vi "Get Message HasOneof.vi"(8 "error in (no error)":errorcluster, 11 "Message ref in":u64) -> (0 "error out":errorcluster, 2 "Has Oneof?":bool, 3 "Message ref out":u64)   [LabVIEW 2019, in "gRPC Template Creation Utility.lvlib"]
uses:
  gRPC Template Creation Utility.lvlib
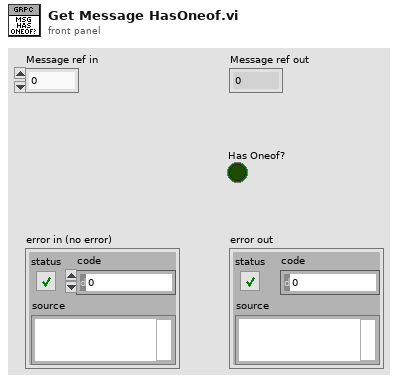
[diagram p1: front panel]
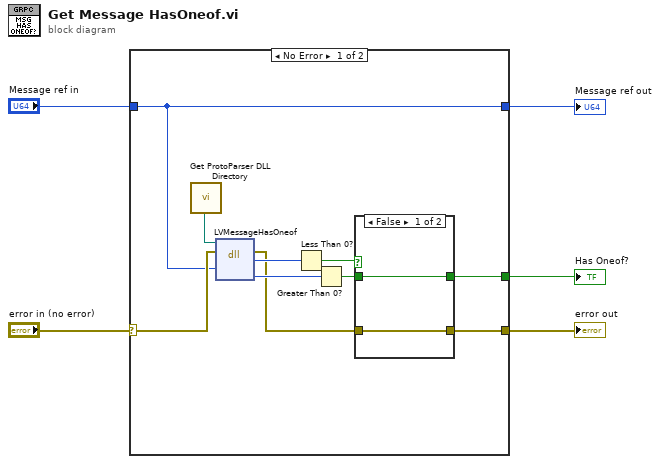
[diagram p0: block diagram]
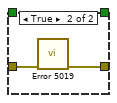
[diagram p2: hidden frame]
diagram:
  n1 = case shown="No Error" "error in (no error)" {
    selector: "error in (no error)" -> [w14 w21]
    tunnel: "Message ref in" -> [w13 w20]
    tunnel: [w13 w20] -> w3
    tunnel: [w7 w21] -> w2
    tunnel: [w11 _] -> w1
    frame No Error {
      n2 = call "Get ProtoParser DLL Directory.vi"() -> ("Proto Parser Directory"=w15:path)
      n3 = dll-call lib="C:/Source/grpc-labview/build/Debug/labview_grpc_generator.dll" fn="LVMessageHasOneof"(path in=w15, error in=w14, "message"=w13) -> (error out=w8:errorcluster, "return type"=w10:i32, "has oneof?"=w12:i32)  [unwired: 3 in, 1 out]
      n4 = Less Than 0?(x=w10) -> (x < 0?=w9:bool)
      n5 = Greater Than 0?(x=w12) -> (x > 0?=w6:bool)
      n6 = case shown="False" w9 {
        tunnel: w6 -> [w16 _]
        tunnel: [w16 _] -> w11
        tunnel: w8 -> [w17 w19]
        tunnel: [w17 w18] -> w7
        frame False {
        }
        frame True {
          n7 = call "Error 5019.vi"("error in (no error)"=w19) -> ("error out"=w18:errorcluster)  [unwired: 10 in]
        }
      }
    }
    frame Error {
    }
  }
  "Message ref out" <- w3
  "error out" <- w2
  "Has Oneof?" <- w1
